vi "Write Observables to string.vi"(1 "Observables":T1[](array[typedef]) {"Weight" min=0.0 max=1.0}) -> (0 "String":string)   [LabVIEW 2020, in "CIRCUS_uServices.lvlib" / "Run Utilities.lvlib" / "Optimiser Cell.lvclass"]
uses:
  Optimiser Cell.lvclass
  Optimisation observable.ctl
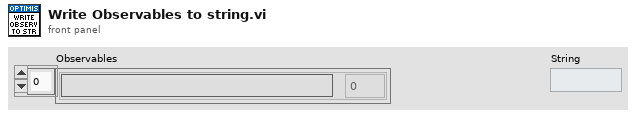
[diagram p1: front panel]
types:
  T1 = typedef "CIRCUS_uServices.lvlib/Run Utilities.lvlib/Optimiser Cell.lvclass/Optimisation observable.ctl" = cluster{"Name":string, "Weight":dbl}
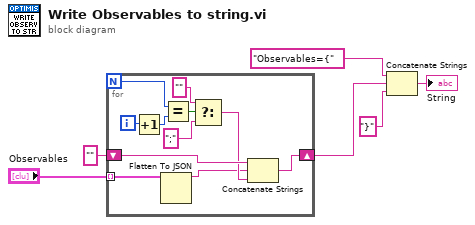
[diagram p0: block diagram]
diagram:
  n1 = for {
    N -> [w13]
    tunnel: "Observables" -> [w8] mode=indexing
    shift-right: [w16] -> w4
    shift-left: "" -> [w17]
    i -> [w15]
    n2 = Increment(x=w15) -> (x+1=w14:i32)
    n3 = Flatten To JSON(anything=w8) -> (JSON string=w7:string)  [unwired: 2 in, 1 out]
    n4 = Equal?(x=w13, y=w14) -> (x = y?=w12:bool)
    n5 = Select(t="" ("string"), s=w12, f=";") -> (s? t:f=w9:string)
    n6 = Concatenate Strings(w17, w7, w9) -> (w16:string)
  }
  n7 = Concatenate Strings("Observables={" ("string"), w4, "}" ("string")) -> (→"String":string)
